vi "close.vi"(8 "error in (no error)":errorcluster, 11 "Stimulus in":refnum<class "Stimulus.lvclass">) -> (0 "error out":errorcluster, 3 "Stimulus out":refnum<class "Stimulus.lvclass">)   [LabVIEW 2014, in "Stimulus.lvclass"]
uses:
  Stimulus.lvclass
  Stimulus.lvclass/Stimulus.ctl
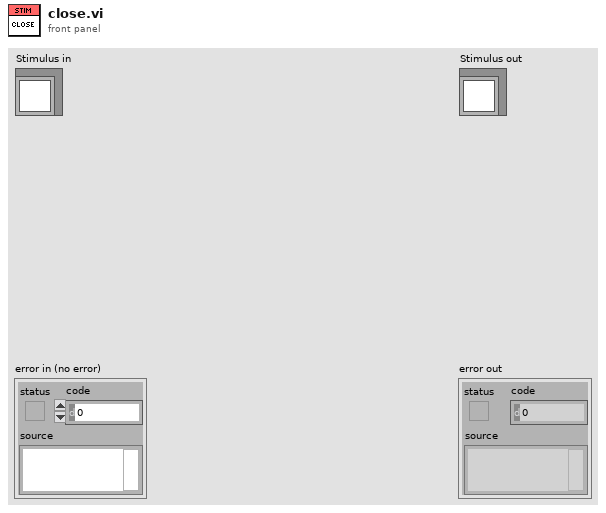
[diagram p1: front panel]
types:
  T1 = typedef "IMAQ Image.ctl" = refnum<image>
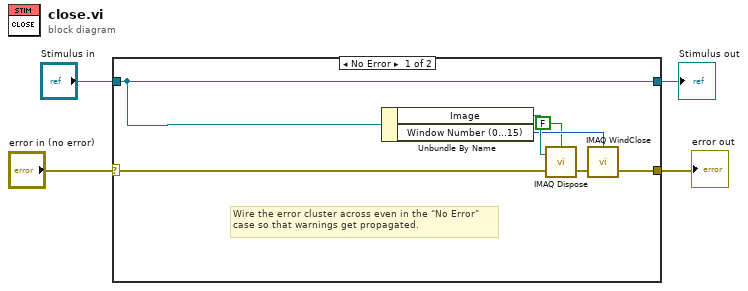
[diagram p0: block diagram]
diagram:
  n1 = case shown="No Error" "error in (no error)" {
    selector: "error in (no error)" -> [w11 w12]
    tunnel: [w10 w12] -> w1
    tunnel: [w6 w13] -> w2
    tunnel: "Stimulus in" -> [w6 w13]
    frame No Error {
      # "Wire the error cluster across even in the \"No Error\"\ncase so that warnings get propagated."
      n2 = Unbundle By Name(w6) -> ("Image"=w8:T1, "Window Number (0...15)"=w7:i32)
      n3 = call "IMAQ Dispose"("All Images? (No)"=FALSE, "Image"=w8, "error in (no error)"=w11) -> ("error out"=w9:errorcluster)  [unwired: 3 in]
      n4 = call "IMAQ WindClose"("Window Number (0...15)"=w7, "error in (no error)"=w9) -> ("error out"=w10:errorcluster)  [unwired: 4 in]
    }
    frame Error {
    }
  }
  "error out" <- w1
  "Stimulus out" <- w2
